vi "TP 1.2.vi"() -> ()   [LabVIEW 2013]
panel:
  out "Boolean 2":bool
  in  "Boolean":bool
  out "String 2":string
  in  "String":string
  out "Numeric 4":i32
  out "Numeric 3":sgl
  in  "Numeric 2":i32
  in  "Numeric":sgl
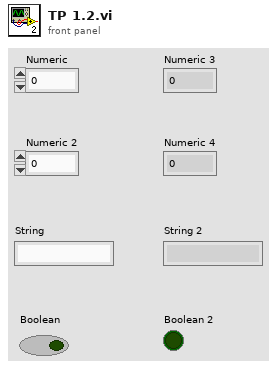
[diagram p1: front panel]
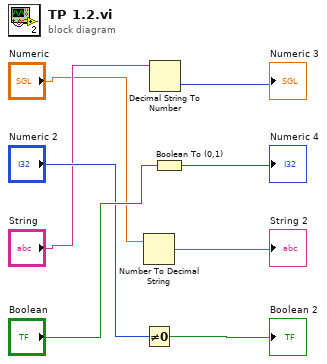
[diagram p0: block diagram]
diagram:
  n1 = Number To Decimal String(number="Numeric") -> (decimal integer string=→"String 2":string)  [unwired: 1 in]
  n2 = Not Equal To 0?(x="Numeric 2") -> (x != 0?=→"Boolean 2":bool)
  n3 = Decimal String To Number(string="String") -> (number=→"Numeric 3":i32)  [unwired: 2 in, 1 out]
  n4 = Boolean To (0,1)(Boolean="Boolean") -> (0, 1=→"Numeric 4":i16)
